vi "量程参数写入.vi"(7 "error in (no error)":errorcluster caption="错误输入（无错误）", 9 "量程参数写入":T1, 10 "测量参数":u16(ring) items=["COD"=22, "氨氮"=3, "总氮"=2, "总磷"=1]) -> (0 "error out":errorcluster caption="错误输出")   [LabVIEW 2022 SP3, in "斯坦道氨氮.lvlib"]
uses:
  <vilib>/Plasmionique/MB Master/MB Master.lvlib
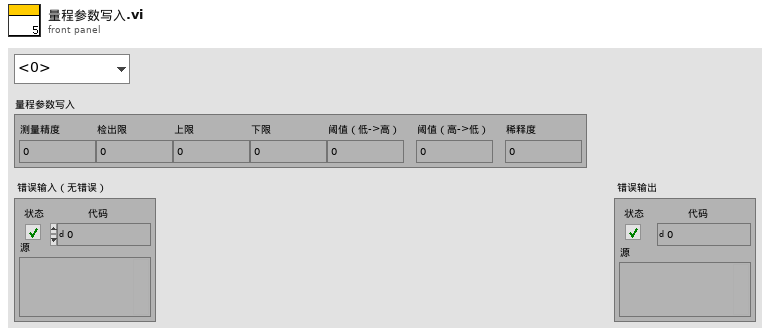
[diagram p1: front panel]
types:
  T1 = cluster{"测量精度":u16, "检出限":dbl, "上限":dbl, "下限":dbl, "阈值（低->高）":dbl, "阈值（高->低）":dbl, "稀释度":dbl}
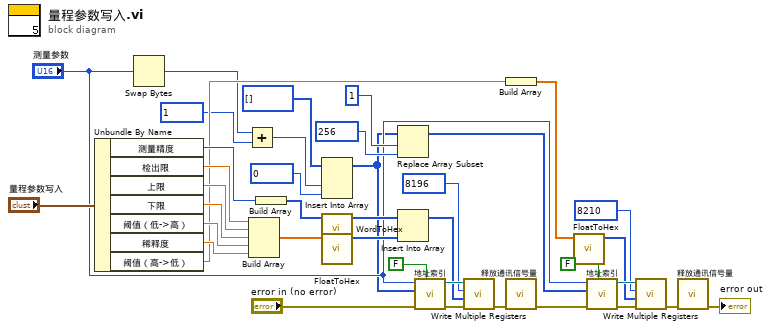
[diagram p0: block diagram]
diagram:
  n1 = Unbundle By Name("量程参数写入") -> ("测量精度"=w34:u16, "检出限"=w33:dbl, "上限"=w32:dbl, "下限"=w31:dbl, "阈值（低->高）"=w30:dbl, "稀释度"=w29:dbl, "阈值（高->低）"=w25:dbl)
  n2 = Swap Bytes(anything="测量参数") -> (byte swapped=w19:u16)
  n3 = Add(x=w19, y=u16 1 ("starting address")) -> (x+y=w23:u16)
  n4 = Build Array(w33, w32, w31, w30, w29) -> (w28:dbl[])
  n5 = Build Array(w34) -> (w35:u16[])
  n6 = Insert Into Array(array=u16[] [] ("数组"), new element #1=w23, new element #2=u16 0 ("starting address")) -> (w9:u16[])  [unwired: 1 in]
  n7 = call "WordToHex.vi"("WORD"=w35) -> ("数组"=w27:u16[])  [unwired: 10 in]
  n8 = call "FloatToHex.vi"("浮点数"=w28) -> ("DCBA整形输出"=w26:u16[])  [unwired: 10 in]
  n9 = Replace Array Subset(array=w9, new element=u16 256 ("starting address"), index=1 ("索引")) -> (w6:u16[])
  n10 = Insert Into Array(array=w27, new element=w26) -> (w7:u16[])  [unwired: 1 in]
  n11 = call "地址索引.vi"("4.2写公式？"=FALSE ("写流程？"), "error in (no error)"="error in (no error)", "values"=w9, "测量参数"="测量参数") -> ("error out"=w17:errorcluster, "MB session out"=w16:refnum<class "MB_Master.lvclass">)  [unwired: 6 in]
  n12 = call <vilib>:"Write Multiple Registers.vi"("error in (no error)"=w17, "values"=w7, "starting address"=u16 8196, "MB session in"=w16) -> ("error out"=w15:errorcluster)  [unwired: 6 in, 1 out]
  n13 = Build Array(w25) -> (w24:dbl[])
  n14 = call "释放通讯信号量.vi"("error in (no error)"=w15) -> ("error out"=w11:errorcluster)  [unwired: 10 in]
  n15 = call "FloatToHex.vi"("浮点数"=w24) -> ("DCBA整形输出"=w4:u16[])  [unwired: 10 in]
  n16 = call "地址索引.vi"("4.2写公式？"=FALSE ("写流程？"), "error in (no error)"=w11, "values"=w6, "测量参数"="测量参数") -> ("error out"=w12:errorcluster, "MB session out"=w13:refnum<class "MB_Master.lvclass">)  [unwired: 6 in]
  n17 = call <vilib>:"Write Multiple Registers.vi"("error in (no error)"=w12, "values"=w4, "starting address"=u16 8210, "MB session in"=w13) -> ("error out"=w14:errorcluster)  [unwired: 6 in, 1 out]
  n18 = call "释放通讯信号量.vi"("error in (no error)"=w14) -> ("error out"=→"error out":errorcluster)  [unwired: 10 in]
